vi "Event Request and Response.vi"(7 "Param (None)":refnum<class>, 8 "error in (no error)":errorcluster, 9 "Timeout mS (-1)":i32=-1, 10 "Response Type":refnum<class>, 11 "Promise Event":refnum<user-event>) -> (0 "error out":errorcluster, 2 "Result":refnum<class>)   [LabVIEW 2020, in "Promises.lvlib" / "Promise.lvclass"]
doc: "Sends an event that has a datatype of Promise and waits for a response via the created Promise. The Promise can optionally send a parameter value so that the request event only needs to handle the promise itself while still transferring other data with the request."
uses:
  Promise.lvclass
  Promise.lvclass/Promise.ctl
  Future/Future.lvclass
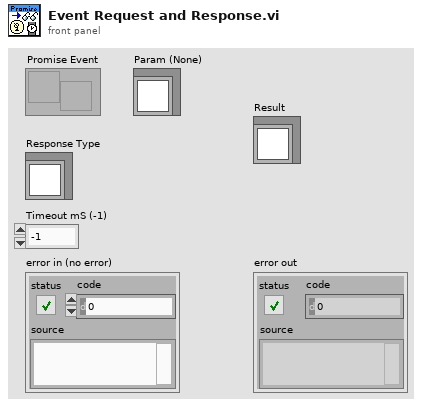
[diagram p1: front panel]
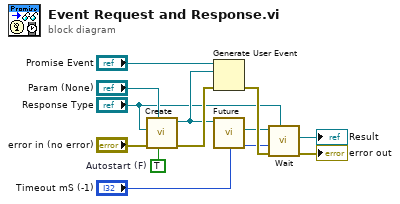
[diagram p0: block diagram]
diagram:
  w10 = TRUE  # Autostart (F)
  n1 = call "Create.vi"("Autostart (F)"=w10, "Param Type (None)"="Param (None)", "error in (no error)"="error in (no error)", "Result Type (None)"="Response Type") -> ("error out"=w11:errorcluster, "Promise"=w3:refnum<class "Promise.lvclass">)  [unwired: 6 in]
  n2 = Generate User Event(user event="Promise Event", event data cluster=w3, error in=w11) -> (error out=w12:errorcluster)  [unwired: 1 in, 1 out]
  n3 = call "Future.vi"("Promise in"=w3) -> ("Future"=w9:refnum<class "Future.lvclass">)  [unwired: 9 in, 1 out]
  n4 = call "Wait.vi"("Result Type"="Response Type", "error in (no error)"=w12, "Timeout mS (-1)"="Timeout mS (-1)", "Future in"=w9) -> ("error out"=→"error out":errorcluster, "Result"=→"Result":refnum<class>)  [unwired: 6 in]
